vi "Spartan HTTP Verify Request.vi"(4 "error in (no error)":errorcluster, 7 "HTTP Data":T4 {"object data"."time" format="%0.2f"}) -> (0 "error out":errorcluster, 2 "request info":T3={"process"=FALSE, "accessed document"="", "request type"=enum."CGI Movie", "reply"={"content"="", "header"="", "keep alive"=FALSE, "don't write"=FALSE}, "script alias"=FALSE}, 3 "dup http session":T4 {"object data"."time" format="%0.2f"})   [LabVIEW 2011]
uses:
  Spartan HTTP Session.ctl
  Addons/internet/http/http_obj.llb/HTTP Session Data.ctl
  Addons/internet/utils/keyedarr.llb/Keyed Array.ctl
  Addons/internet/http/http1.llb/HTTP Request Type.ctl
  Addons/internet/http/cgi.llb/CGI Reply.ctl
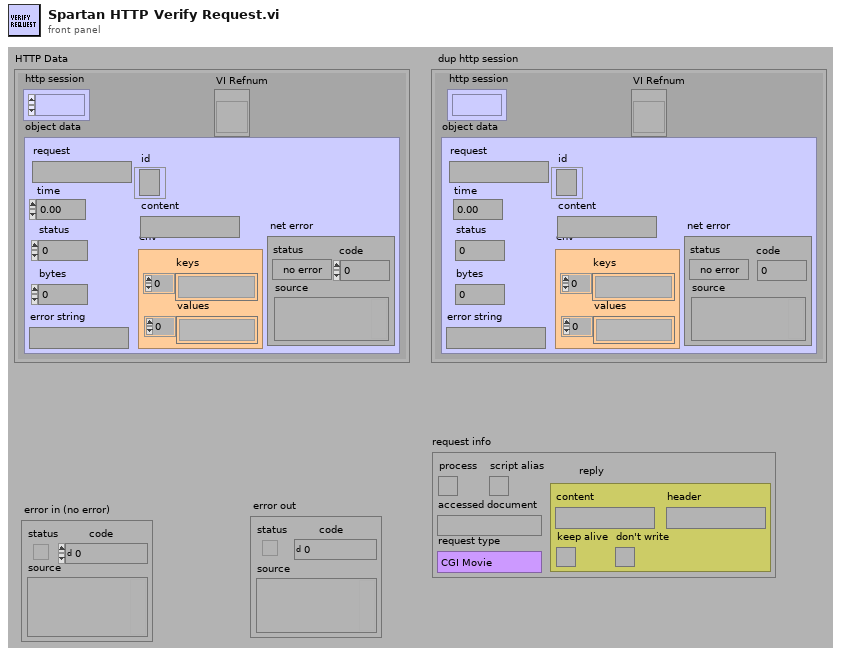
[diagram p1: front panel]
types:
  T1 = typedef "HTTP Request Type.ctl" = enum16{"Default", "Panel Picture", "Panel Movie", "CGI Movie"}
  T2 = typedef "CGI Reply.ctl" = cluster{"content":string, "header":string, "keep alive":bool, "don't write":bool}
  T3 = cluster{"process":bool, "accessed document":string, "request type":T1, "reply":T2, "script alias":bool}
  T4 = typedef "Spartan HTTP Session.ctl" = cluster{"http session":refnum<k1>, "object data":T5, "VI Refnum":refnum<vi>}
  T5 = typedef "HTTP Session Data.ctl" = cluster{"request":string, "time":dbl, "status":i32, "error string":string, "bytes":i32, "env":T6, "content":string, "id":refnum<k5>, "net error":errorcluster}
  T6 = typedef "Keyed Array.ctl" = cluster{"keys":string[], "values":string[]}
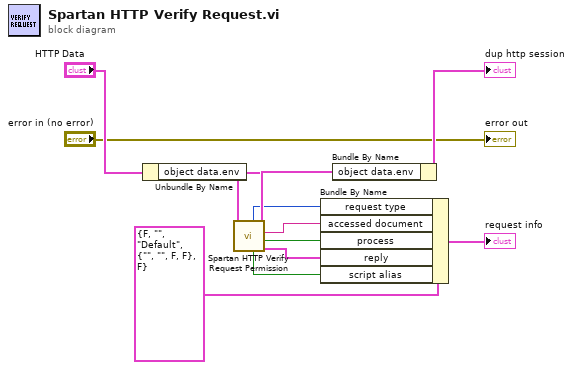
[diagram p0: block diagram]
diagram:
  n1 = Unbundle By Name("HTTP Data") -> ("object data.env"=w11:T6)
  n2 = call "Spartan HTTP Verify Request Permission.vi"("env"=w11) -> ("reply"=w6:T2, "process"=w7:bool, "accessed document"=w4:string, "env out"=w12:T6, "script alias"=w8:bool, "request type"=w5:T1)  [unwired: 5 out]
  n3 = Bundle By Name(cluster=T3 {"process"=FALSE, "accessed document"="", "request type"=enum."Default", "reply"={"content"="", "header"="", "keep alive"=FALSE, "don't write"=FALSE}, "script alias"=FALSE} ("request info"), "request type"=w5, "accessed document"=w4, "process"=w7, "reply"=w6, "script alias"=w8) -> (→"request info":T3)
  n4 = Bundle By Name(cluster="HTTP Data", "object data.env"=w12) -> (→"dup http session":T4)
  "error out" <- "error in (no error)"
